vi "Build DIO_Query query command substring.vi"(0 "System no.":i32=1 min=1 max=4 step=1, 2 "DI's to query in":string[](array[string]), 3 "Query all DI's?":bool, 4 "For all DI's: use\nDI identifier?":bool=TRUE, 5 "error in":errorcluster, 6 "For all DI's: \nInvert order for TVI?":bool=TRUE) -> (14 "Command substring":string, 15 "DI's to query out":string[](array[string]), 16 "Number of rows":u32=1, 19 "error out":errorcluster)   [LabVIEW 2020]
doc: "This VI builds a DIO? query command substring. If Query all DI's is TRUE, available analog inputs are read using TIO? and DI identifiers are assigned using TVI? (valid identifiers are assigned to available DI's in ascending order) (GCS 1.0) or 1 to x with x being the number of available analog inputs (GCS 2.0). Number of rows is the size of the DI's to query out array. If DI identifier is FALSE, command substring is an empty string."
uses:
  Syntax.ctl
  Global1.vi
panel:
  # "This vi builds a DIO? query command substring. If \"Query all DI's\" is true, available analog inputs\nare read using TIO? and DI identifiers are assigned using TVI? (valid identifiers are assigned\nto available DI's in ascending order). \"Number of rows\" is the size of the \"DI's to query out\" array.\nIf \"Use DI identifier\" is false, command substring is an empty string."
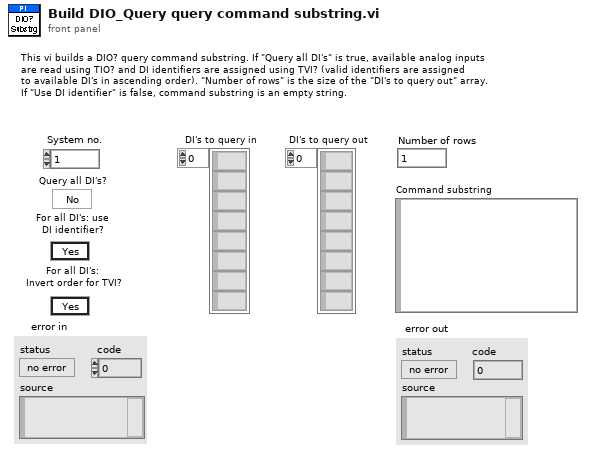
[diagram p1: front panel]
types:
  T1 = typedef "Syntax.ctl" = enum16{"GCS 1.0", "GCS 2.0", "GCS 3.0"}
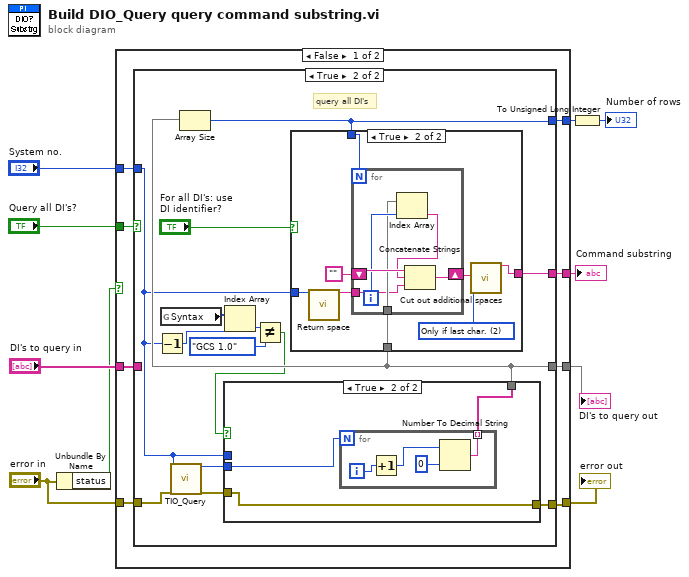
[diagram p0: block diagram]
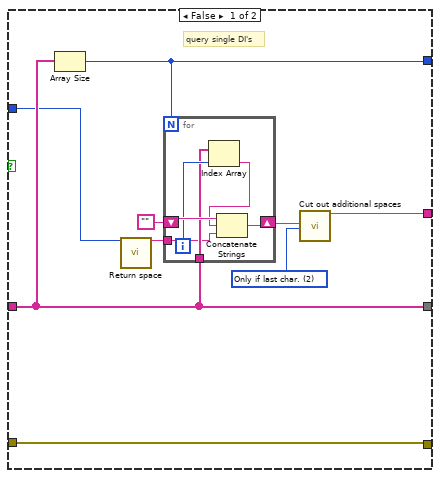
[diagram p2: hidden frame]
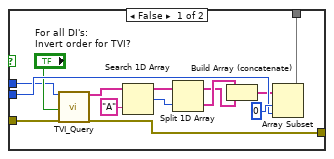
[diagram p3: hidden frame]
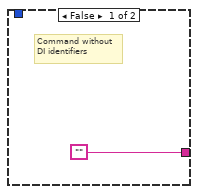
[diagram p4: hidden frame]
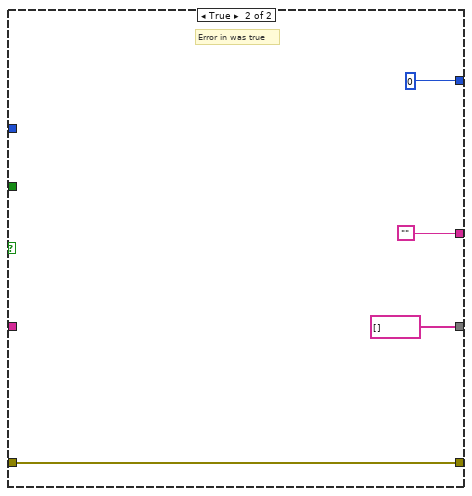
[diagram p5: hidden frame]
diagram:
  n1 = Unbundle By Name("error in") -> ("status"=w5:bool)
  n2 = case shown="False" w5 {
    tunnel: [w18 0] -> w10
    tunnel: "DI's to query in" -> [w17 _]
    tunnel: "Query all DI's?" -> [w16 _]
    tunnel: [w15 string[] [] ("Relais to query in")] -> w7
    tunnel: [w14 ""] -> w6
    tunnel: [w12 w86] -> w4
    tunnel: "error in" -> [w13 w86]
    tunnel: "System no." -> [w11 _]
    frame False {
      n3 = case shown="True" w16 {
        tunnel: [w22 w47] -> w14
        tunnel: w17 -> [w21 _]
        tunnel: [w21 w41] -> w15
        tunnel: [w20 w46] -> w18
        tunnel: w13 -> [w27 w44]
        tunnel: [w27 w42] -> w12
        tunnel: w11 -> [w19 w36]
        frame False {
          w24 = u16 2 items=["All Spaces", "Only if 1st char.", "Only if last char.", "Only if near \"=\"", "Only if 1st or last char.", "Only multiple"] ("Mode")
          # "query single DI's"
          n4 = Array Size(array=w21) -> (size(s)=w20:i32)
          n5 = call "Return space.vi"("System no."=w19) -> ("String out"=w23:string)  [unwired: 1 in, 17 out]
          n6 = for {
            N: w20 -> [_]
            shift-right: [w32] -> w25
            shift-left: "" -> [w33]
            tunnel: w21 -> [w30]
            tunnel: w23 -> [w28]
            i -> [w31]
            n7 = Index Array(array=w30, index=w31) -> (element=w29:string)
            n8 = Concatenate Strings(w33, w29, w28) -> (w32:string)
          }
          n9 = call "Cut out additional spaces.vi"("String"=w25, "Mode"=w24) -> ("String out"=w22:string)  [unwired: 17 out]
        }
        frame True {
          # "query all DI's"
          n10 = Decrement(x=w36) -> (x-1=w38:i32)
          n11 = global read "Global1.vi" "Syntax"() -> (w37:T1[])
          n12 = call "TIO_Query.vi"("System no."=w36, "error in"=w44) -> ("No. of dig. inputs"=w40:i32, "error out"=w43:errorcluster)  [unwired: 16 out]
          n13 = Index Array(array=w37, index=w38) -> (element=w39:T1)
          n14 = Not Equal?(x=w39, y=Syntax."GCS 1.0") -> (x != y?=w35:bool)
          n15 = case shown="True" w35 {
            tunnel: w43 -> [w60 w63]
            tunnel: [w59 w63] -> w42
            tunnel: [w57 w61] -> w41
            tunnel: w40 -> [w56 w62]
            tunnel: w36 -> [w48 _]
            frame False {
              n16 = call "TVI_Query.vi"("System no."=w48, "Invert order"="For all DI's: \nInvert order for TVI?", "error in"=w60) -> ("Valid axis IDs"=w51:string[], "error out"=w59:errorcluster)  [unwired: 15 out]
              n17 = Search 1D Array(1D array=w51, element="A") -> (index of element=w54:i32)  [unwired: 1 out]
              n18 = Split 1D Array(array=w51, index=w54) -> (first subarray=w52:string[], second subarray=w53:string[])
              n19 = Build Array (concatenate)(w53, w52) -> (w50:string[])
              n20 = Array Subset(array=w50, index=0 ("Array Index"), length=w56) -> (w57:string[])
            }
            frame True {
              n21 = for {
                N: w62 -> [_]
                tunnel: [w64] -> w61 mode=indexing
                i -> [w67]
                n22 = Increment(x=w67) -> (x+1=w66:i32)
                n23 = Number To Decimal String(number=w66, width (-)=i16 0) -> (decimal integer string=w64:string)
              }
            }
          }
          n24 = Array Size(array=w41) -> (size(s)=w46:i32)
          n25 = case shown="True" "For all DI's: use\nDI identifier?" {
            tunnel: ["" w72] -> w47
            tunnel: w41 -> [_ w76]
            tunnel: w46 -> [_ w74]
            tunnel: w36 -> [_ w69]
            frame False {
              # "Command without\nDI identifiers"
            }
            frame True {
              w71 = u16 2 items=["All Spaces", "Only if 1st char.", "Only if last char.", "Only if near \"=\"", "Only if 1st or last char.", "Only multiple"] ("Mode")
              n26 = call "Return space.vi"("System no."=w69) -> ("String out"=w70:string)  [unwired: 1 in, 17 out]
              n27 = for {
                N: w74 -> [_]
                shift-right: [w81] -> w73
                shift-left: "" -> [w82]
                tunnel: w76 -> [w79]
                tunnel: w70 -> [w77]
                i -> [w80]
                n28 = Index Array(array=w79, index=w80) -> (element=w78:string)
                n29 = Concatenate Strings(w82, w78, w77) -> (w81:string)
              }
              n30 = call "Cut out additional spaces.vi"("String"=w73, "Mode"=w71) -> ("String out"=w72:string)  [unwired: 17 out]
            }
          }
        }
      }
    }
    frame True {
      # "Error in was true"
    }
  }
  "DI's to query out" <- w7
  "Command substring" <- w6
  "error out" <- w4
  n31 = To Unsigned Long Integer(number=w10) -> (unsigned 32bit integer=→"Number of rows":u32)
